vi "4장.vi"() -> ()   [LabVIEW 2014]
panel:
  in  "불리언 2":bool
  in  "불리언":bool
  in  "노브":dbl(knob) scale=0.0..10.0
  out "라벨.텍스트":string
  in  "구매":bool
  out "숫자형 2":dbl
  in  "숫자형":dbl
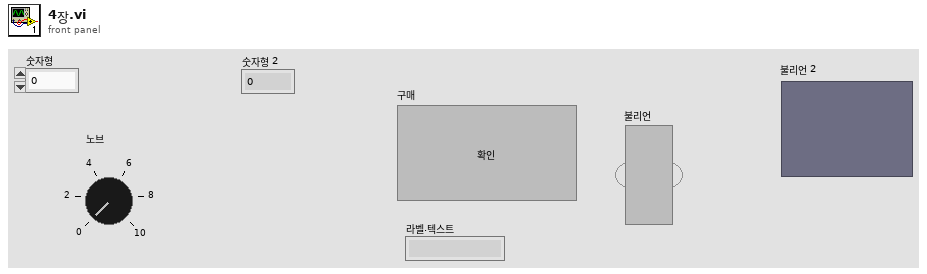
[diagram p1: front panel]
types:
  T1 = enum8{"Enabled", "Disabled", "Disabled and Grayed Out"}
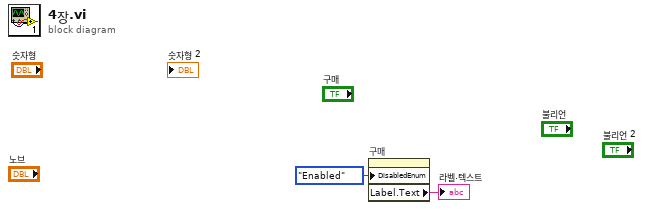
[diagram p0: block diagram]
diagram:
  n1 = property on="구매" class="Bool"("DisabledEnum"=T1."Enabled" ("비활성화")) -> ("Label.Text"=→"라벨.텍스트":string)  [unwired: 2 in, 2 out]
